vi "Generate Signal.vi"(8 "error in (no error)":errorcluster, 9 "Amplitude (1)":dbl=1.0, 10 "Frequency (1000 Hz)":dbl=1000.0, 11 "Simulated Sig Gen in":refnum<class "Simulated Sig Gen.lvclass">) -> (0 "error out":errorcluster, 3 "Simulated Sig Gen out":refnum<class "Simulated Sig Gen.lvclass">)   [LabVIEW 2011, in "Simulated Sig Gen.lvclass"]
uses:
  Simulated Sig Gen.lvclass
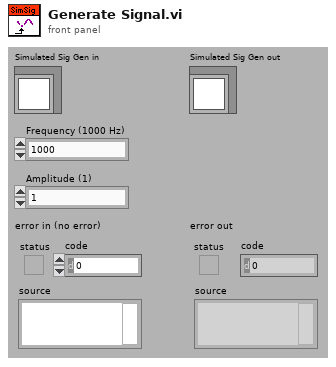
[diagram p1: front panel]
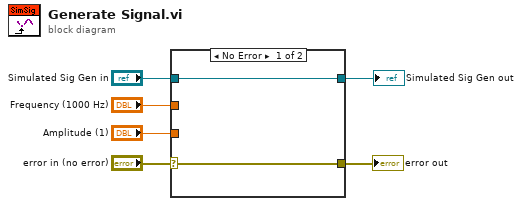
[diagram p0: block diagram]
diagram:
  n1 = case shown="No Error" "error in (no error)" {
    selector: "error in (no error)" -> [w7 w9]
    tunnel: "Simulated Sig Gen in" -> [w8 w10]
    tunnel: [w8 w10] -> w5
    tunnel: [w7 w9] -> w4
    tunnel: "Frequency (1000 Hz)" -> [_ _]
    tunnel: "Amplitude (1)" -> [_ _]
    frame No Error {
    }
    frame Error {
    }
  }
  "error out" <- w4
  "Simulated Sig Gen out" <- w5
